vi "Bool to string.vi"(11 "Boolean":bool) -> (3 "0/1":string, 5 "int_0, 1":i16)   [LabVIEW 2021]
doc: "bool to 0 or 1 string"
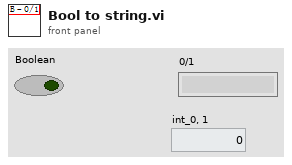
[diagram p1: front panel]
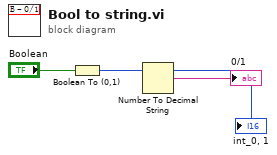
[diagram p0: block diagram]
diagram:
  n1 = Boolean To (0,1)(Boolean="Boolean") -> (0, 1=w2:i16)
  "int_0, 1" <- w2
  n2 = Number To Decimal String(number=w2) -> (decimal integer string=→"0/1":string)  [unwired: 1 in]
